vi "readPressureSensor.vi"(8 "error in (no error)":errorcluster, 11 "Model in":refnum<class "Model.lvclass">) -> (0 "error out":errorcluster, 3 "Model out":refnum<class "Model.lvclass">)   [LabVIEW 2015]
uses:
  PressureSensor/PressureSensor/PressureSensor.lvclass
  Model.lvclass
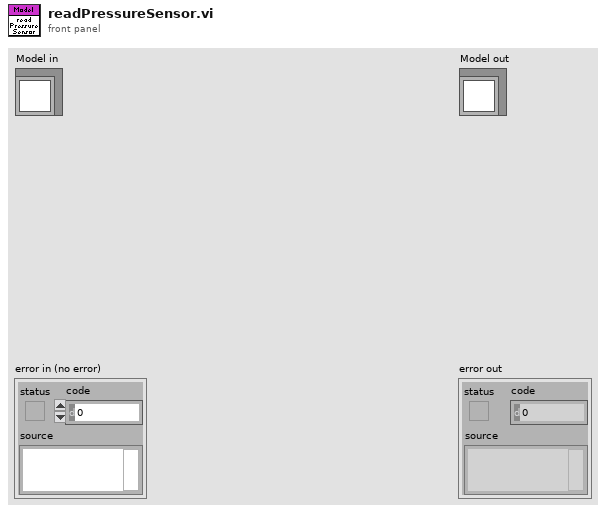
[diagram p1: front panel]
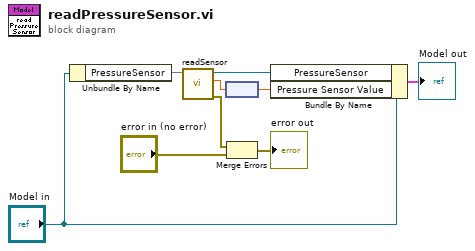
[diagram p0: block diagram]
diagram:
  n1 = Unbundle By Name("Model in") -> ("PressureSensor"=w7)
  n2 = call "readSensor.vi"("PressureSensor in"=w7) -> ("error out"=w5:errorcluster, "Pressure Sensor 1"=w1:dbl, "PressureSensor out"=w6:refnum<class "PressureSensor.lvclass">)  [unwired: 8 in]
  n3 = node(w1) -> (w2:dbl[unit])
  n4 = Merge Errors(w5, "error in (no error)") -> (→"error out":errorcluster)
  n5 = Bundle By Name(cluster="Model in", "PressureSensor"=w6, "Pressure Sensor Value"=w2) -> (→"Model out":cluster{})
